vi "测试-模式插入节点.vi"() -> ()   [LabVIEW 2019]
panel:
  in  "确定按钮":bool
  in  "停止":bool
  in  "按键编号":string
  in  "模式input":T1
  in  "动作":string(combo)
  in  "按键名字":string(combo)
  in  "面板地址":string(combo)
  in  "模式选择":string(combo)
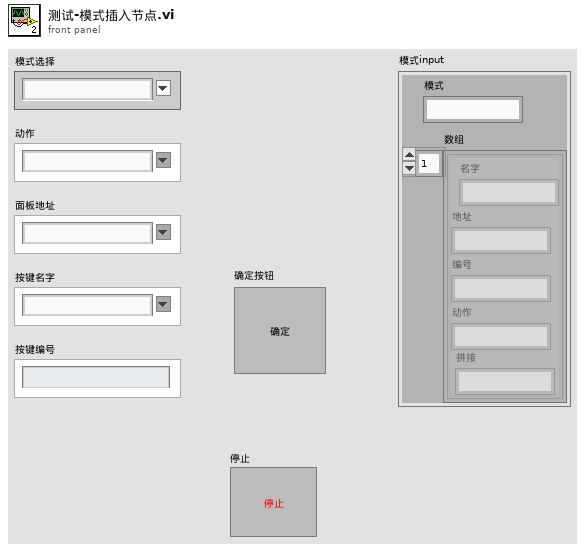
[diagram p1: front panel]
types:
  T1 = cluster{"模式":string, "数组":cluster{"地址":string, "名字":string, "编号":string, "动作":string, "拼接":string}[]}
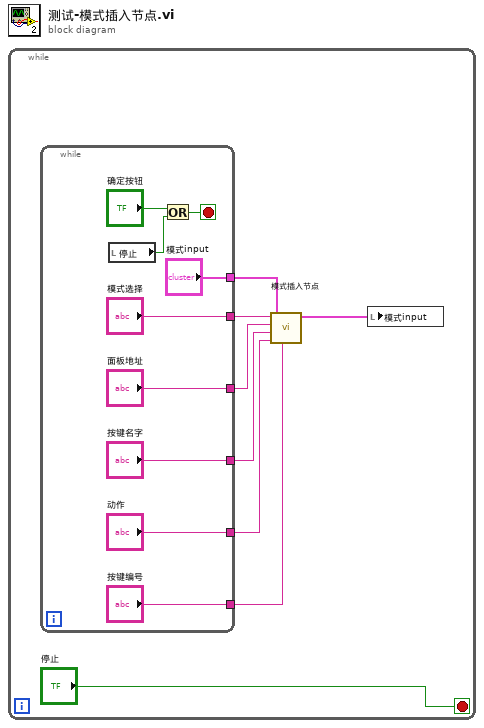
[diagram p0: block diagram]
diagram:
  n1 = while {
    stop <- "停止" stop-if-true
    n2 = while {
      tunnel: ["按键编号"] -> w7
      tunnel: ["动作"] -> w6
      tunnel: ["按键名字"] -> w5
      tunnel: ["面板地址"] -> w4
      tunnel: ["模式选择"] -> w3
      tunnel: ["模式input"] -> w1
      stop <- w17 stop-if-true
      n3 = local read "停止"() -> (w16:bool)
      n4 = Or(x="确定按钮", y=w16) -> (x .or. y?=w17:bool)
    }
    n5 = call "模式插入节点.vi"("按键编号"=w7, "模式input"=w1, "动作"=w6, "按键名字"=w5, "面板地址"=w4, "模式选择"=w3) -> ("模式output"=w2:T1)  [unwired: 5 in]
    n6 = local write "模式input"(w2) -> ()
  }
